vi "Configure IF Bandwith.vi"(8 "error in (no error)":errorcluster, 10 "IF BW [Hz]":dbl, 11 "VNA-ENA in":refnum<class "VNA-ENA.lvclass">) -> (0 "error out":errorcluster, 2 "IF BW used [Hz]":dbl, 3 "VNA-ENA out":refnum<class "VNA-ENA.lvclass">)   [LabVIEW 2020, in "VNA-ENA.lvclass"]
doc: "Configures the Intermidiate Frequency Bandwidth. \nIt chooses the closest supported bandwidth.\nIt returns the used IF BW."
uses:
  VNA-ENA.lvclass
  C:/Sandbox/Git_Sandbox/WiSpry Test Framework source code (LV20)/WiSpry Test Framework/Instruments/Instrument.lvclass
  Instrument.lvclass/Instrument.ctl
  Instrument.lvclass
  <instrlib>/Agilent ENA Series/Agilent ENA Series.lvlib
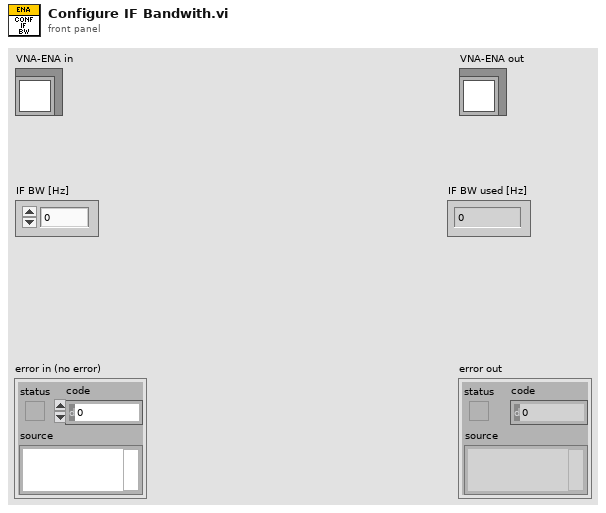
[diagram p1: front panel]
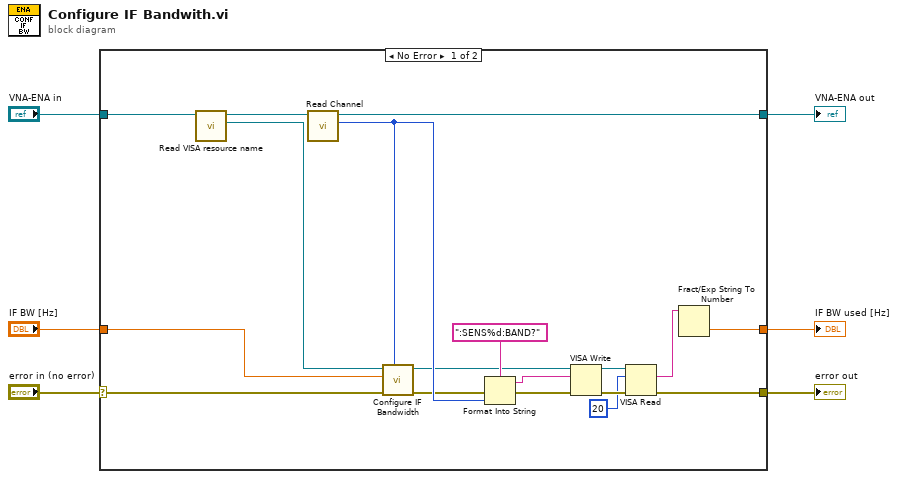
[diagram p0: block diagram]
diagram:
  n1 = case shown="No Error" "error in (no error)" {
    selector: "error in (no error)" -> [w23 w27]
    tunnel: [w15 w27] -> w3
    tunnel: [w18 w26] -> w4
    tunnel: "VNA-ENA in" -> [w24 w26]
    tunnel: "IF BW [Hz]" -> [w21 w25]
    tunnel: [w7 w25] -> w1
    frame No Error {
      n2 = call "Read VISA resource name.vi"("Instrument in"=w24) -> ("VISA resource name"=w22:refnum<visa-resource-name>, "Instrument out"=w19:refnum<class "VNA-ENA.lvclass">)  [unwired: 9 in]
      n3 = call-dynamic "Read Channel.vi"("Vector Network Analyzer in"=w19) -> ("Channel"=w17:i32, "Vector Network Analyzer out"=w18:refnum<class "VNA-ENA.lvclass">)  [unwired: 9 in]
      n4 = call <instrlib>:"Configure IF Bandwidth.vi"("Channel (1)"=w17, "error in (no error)"=w23, "IF Bandwidth (100000.0)"=w21, "VISA resource name"=w22) -> ("error out"=w16:errorcluster, "VISA resource name out"=w12:refnum<visa-resource-name>)  [unwired: 6 in]
      n5 = Format Into String(format string=":SENS%d:BAND?", error in=w16, w17) -> (resulting string=w10:string, error out=w11:errorcluster)  [unwired: 1 in]
      n6 = VISA Write(VISA resource name=w12, write buffer=w10, error in (no error)=w11) -> (VISA resource name out=w13:refnum<visa-resource-name>, error out=w14:errorcluster)  [unwired: 1 out]
      n7 = VISA Read(VISA resource name=w13, byte count=u32 20, error in (no error)=w14) -> (read buffer=w8:string, error out=w15:errorcluster)  [unwired: 2 out]
      n8 = Fract/Exp String To Number(string=w8) -> (number=w7:dbl)  [unwired: 3 in, 1 out]
    }
    frame Error {
    }
  }
  "error out" <- w3
  "VNA-ENA out" <- w4
  "IF BW used [Hz]" <- w1
